vi "RunProgram.vi"(1 "Program":path=path "C:/FingerPressRT.exe", 2 "IpAddress":string="155.101.184.62", 3 "Mode":enum16{"Start", "Stop"}(ring)=enum."Stop") -> (0 "standard output":string="\r\nGAC    Version        Location                                                 \r\n---    -------        --------                                                 \r\nTrue   v2.0.50727     C:\\Windows\\assembly\\GAC_MSIL\\Microsoft.VisualBasic\\8.0...\r\nprocessid: \nresult: 0\n\r\n\r\n")   [LabVIEW 2011]
panel:
  out "ProgStr":string="C:\\temp\\notepad.exe"
  out "standard error":string
  out "Result":string="0"
  out "ProcessId":string
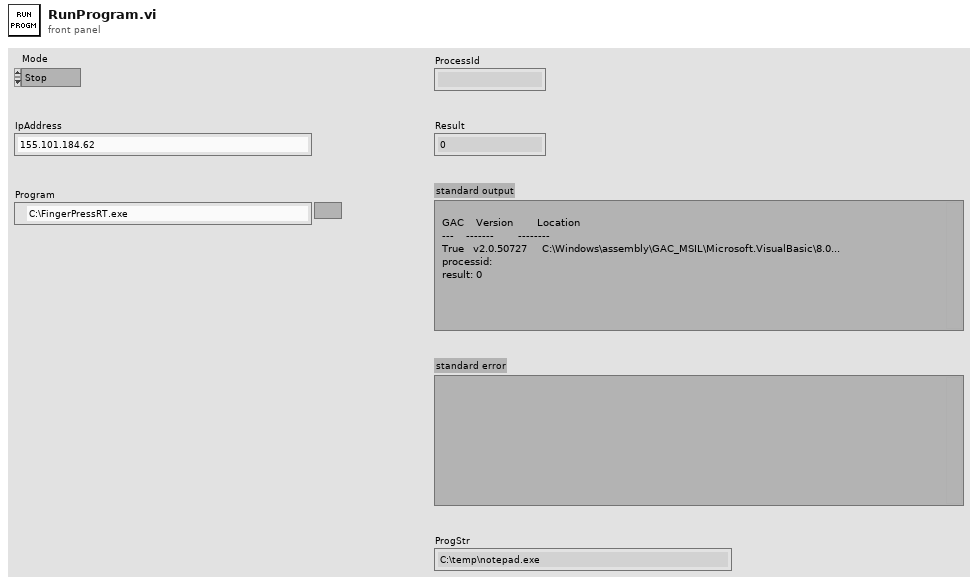
[diagram p1: front panel]
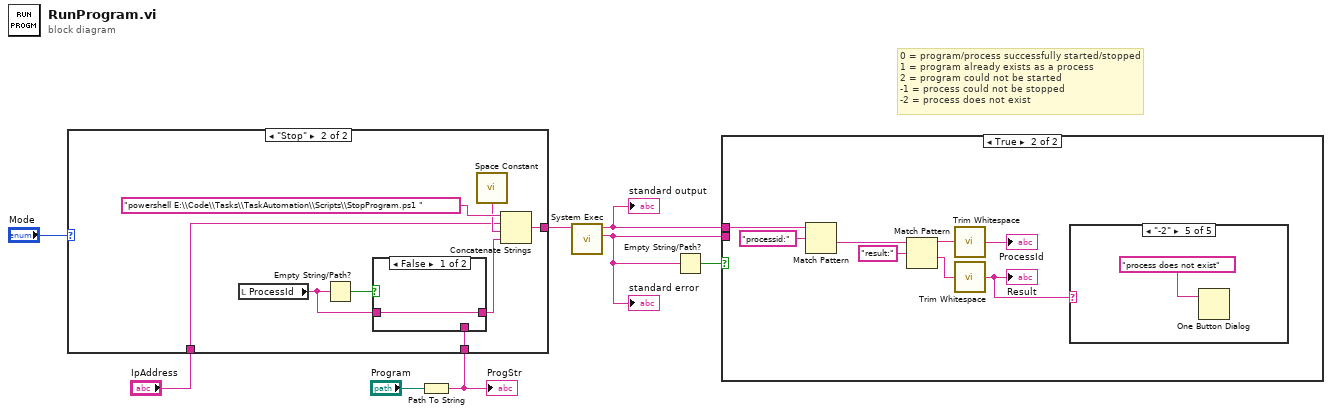
[diagram p0: block diagram]
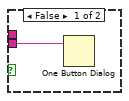
[diagram p2: hidden frame]
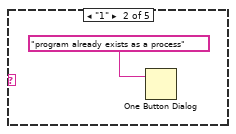
[diagram p4: hidden frame]
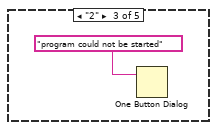
[diagram p5: hidden frame]
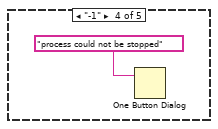
[diagram p6: hidden frame]
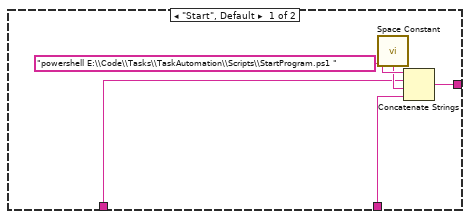
[diagram p7: hidden frame]
diagram:
  # "0 = program/process successfully started/stopped\n1 = program already exists as a process\n2 = program could not be started\n-1 = process could not be stopped\n-2 = process does not exist"
  n1 = Path To String(path="Program") -> (string=w1:string)
  "ProgStr" <- w1
  n2 = case shown="\"Stop\"" "Mode" {
    tunnel: [w12 w19] -> w8
    tunnel: "IpAddress" -> [w10 w15]
    tunnel: w1 -> [w9 w14]
    frame "Start", Default {
      n3 = call <vilib>:"Space Constant.vi"() -> ("String"=w11:string)
      n4 = Concatenate Strings("powershell E:\\Code\\Tasks\\TaskAutomation\\Scripts\\StartProgram.ps1 " ("command line"), w10, w11, w9) -> (w12:string)
    }
    frame "Stop" {
      n5 = local read "ProcessId"() -> (w17:string)
      n6 = Empty String/Path?(string/path=w17) -> (empty?=w18:bool)
      n7 = case shown="False" w18 {
        tunnel: w17 -> [w22 _]
        tunnel: [w22 w23] -> w16
        tunnel: w14 -> [_ w23]
        frame False {
        }
        frame True {
        }
      }
      n8 = call <vilib>:"Space Constant.vi"() -> ("String"=w20:string)
      n9 = Concatenate Strings("powershell E:\\Code\\Tasks\\TaskAutomation\\Scripts\\StopProgram.ps1 " ("command line"), w15, w20, w16) -> (w19:string)
    }
  }
  n10 = call <vilib>:"System Exec.vi"("command line"=w8) -> ("standard error"=w4:string, "standard output"=w7:string)  [unwired: 7 in, 2 out]
  "standard output" <- w7
  "standard error" <- w4
  n11 = Empty String/Path?(string/path=w4) -> (empty?=w5:bool)
  n12 = case shown="True" w5 {
    tunnel: w7 -> [_ w32]
    tunnel: w4 -> [w24 _]
    frame False {
      n13 = One Button Dialog(message=w24) -> ()  [unwired: 1 in, 1 out]
    }
    frame True {
      n14 = Match Pattern(string=w32, regular expression="processid:") -> (after substring=w30:string)  [unwired: 1 in, 3 out]
      n15 = Match Pattern(string=w30, regular expression="result:") -> (before substring=w28:string, after substring=w27:string)  [unwired: 1 in, 2 out]
      n16 = call <vilib>:"Trim Whitespace.vi"("string"=w28) -> ("trimmed string"=→"ProcessId":string)  [unwired: 1 in]
      n17 = call <vilib>:"Trim Whitespace.vi"("string"=w27) -> ("trimmed string"=w26:string)  [unwired: 1 in]
      "Result" <- w26
      n18 = case shown="\"-2\"" w26 {
        frame "0", Default {
        }
        frame "1" {
          n19 = One Button Dialog(message="program already exists as a process") -> ()  [unwired: 1 in, 1 out]
        }
        frame "2" {
          n20 = One Button Dialog(message="program could not be started") -> ()  [unwired: 1 in, 1 out]
        }
        frame "-1" {
          n21 = One Button Dialog(message="process could not be stopped") -> ()  [unwired: 1 in, 1 out]
        }
        frame "-2" {
          n22 = One Button Dialog(message="process does not exist") -> ()  [unwired: 1 in, 1 out]
        }
      }
    }
  }
